vi "sub_main_vision.vi"(8 "error in":errorcluster) -> (0 "error out":errorcluster)   [LabVIEW 2019]
uses:
  <vilib>/vision/NI_Vision_Development_Module.lvlib
panel:
  out "강도 그래프":u8[][](graph)
  out "Image Pixels (U8)":u8[][](array[numeric])
  in  "Replace Value":sgl=1.0 format="%.2f"
  out "loop":i32
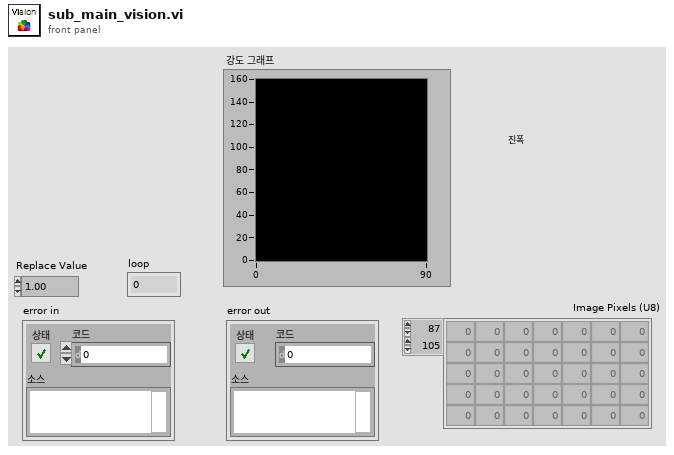
[diagram p1: front panel]
types:
  T1 = enum16{"none", "C920", "C922", "GT1290C", "MS LifeCam"}
  T2 = typedef "system_hw.ctl" = cluster{"AGV":enum16{"none", "ERP42", "ERP42mini", "Scout", "Ycar"}, "Lidar 1":enum16{"none", "VLP16", "TIM571", "RPLidar A2", "RPLidar A3"}, "Lidar 2":enum16{"none", "VLP16", "TIM571", "RPLidar A2", "RPLidar A3"}, "GPS":enum16{"none", "F9P", "M8P", "PwrPak7", "19X HVS"}, "Camera":enum16{"none", "C920", "C922", "GT1290C", "MS LifeCam"}, "Joystick":enum16{"none", "joystick"}}
  T3 = typedef "IMAQ Image.ctl" = refnum<image>
  T4 = cluster{"Clamp Settings":cluster{"Contrast":i32, "Filter width":i32, "Steepness":i32, "Subsampling Ratio":u32, "Show Search Area":bool, "Show Search Lines":bool, "Show Edges Found":bool, "Show Result":bool}, "Range":cluster{"Lower value":sgl, "Upper value":sgl}, "N of Erosion 1":i32, "N of Erosion 2":i32}
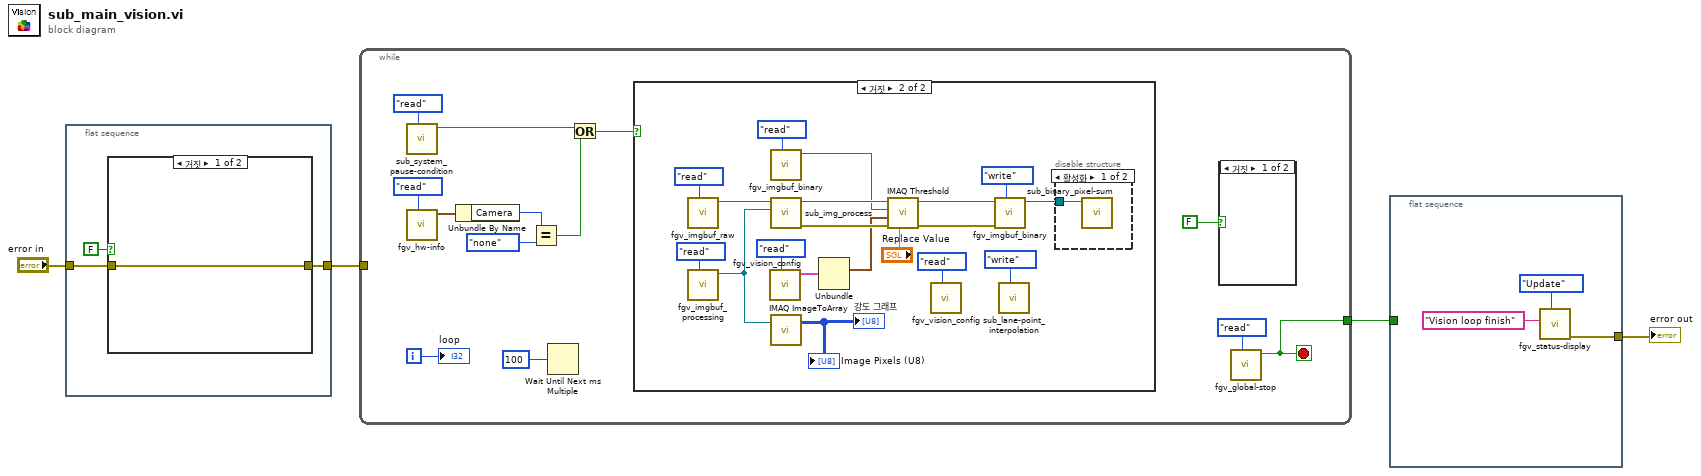
[diagram p0: block diagram]
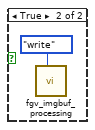
[diagram p2: hidden frame]
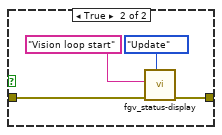
[diagram p5: hidden frame]
diagram:
  n1 = flat-sequence {
    tunnel: "error in" -> [w7]
    tunnel: [w6] -> w4
    frame #0 {
      n2 = case shown="거짓" FALSE {
        tunnel: w7 -> [w8 w10]
        tunnel: [w8 w9] -> w6
        frame False {
        }
        frame True {
          n3 = call "fgv_status-display.vi"("Mode"=enum16{"Initial", "Update", "Clear"}."Update", "error in"=w10, "title"="Vision loop start" ("String in 1")) -> ("error out"=w9:errorcluster)  [unwired: 8 in]
        }
      }
    }
  }
  n4 = while {
    tunnel: [w24] -> w1
    tunnel: w4 -> [_]
    i -> [w21]
    stop <- w24 stop-if-true
    n5 = call "sub_system_pause-condition.vi"("cmd"=enum16{"pause", "go", "read"}."read") -> ("pause"=w14:bool)  [unwired: 10 in]
    n6 = call "fgv_hw-info.vi"("cmd"=enum16{"write", "read"}."read") -> ("HW info out"=w18:T2)  [unwired: 10 in]
    n7 = Unbundle By Name(w18) -> ("Camera"=w17:T1)
    n8 = Equal?(x=w17, y=T1."none") -> (x = y?=w15:bool)
    n9 = Wait Until Next ms Multiple(millisecond multiple=u32 100 ("dt")) -> ()  [unwired: 1 out]
    n10 = Or(x=w14, y=w15) -> (x .or. y?=w13:bool)
    n11 = case shown="거짓" w13 {
      frame True {
      }
      frame False {
        n12 = call "fgv_imgbuf_raw.vi"("cmd"=enum16{"create", "close", "write", "read"}."read") -> ("Image"=w43:T3)  [unwired: 9 in, 1 out]
        n13 = call "fgv_imgbuf_processing.vi"("cmd"=enum16{"create", "close", "write", "read"}."read") -> ("Image"=w29:T3)  [unwired: 9 in, 1 out]
        n14 = call "fgv_vision_config.vi"("cmd"=enum16{"init", "read", "write"}."read") -> ("Vison cfg out"=w37:T4)  [unwired: 9 in, 1 out]
        n15 = call "fgv_imgbuf_binary.vi"("cmd"=enum16{"create", "close", "write", "read"}."read") -> ("raw image out"=w31:T3)  [unwired: 9 in, 1 out]
        n16 = call "sub_img_process.vi"("Green or Sat Plane"=w29, "Image Src"=w43) -> ("error out"=w39:errorcluster, "Image Dst Out"=w41:T3)  [unwired: 8 in]
        n17 = call "IMAQ ImageToArray"("Image"=w29) -> ("Image Pixels (U8)"=→"Image Pixels (U8)" →"강도 그래프":u8[][])  [unwired: 3 in, 4 out]
        n18 = Unbundle(w37) -> ("Range"=w35:cluster{"Lower value":sgl, "Upper value":sgl})  [unwired: 3 out]
        n19 = call "IMAQ Threshold"("Replace Value"="Replace Value", "error in (no error)"=w39, "Range"=w35, "Image Dst"=w31, "Image Src"=w41) -> ("error out"=w27:errorcluster, "Image Dst Out"=w28:T3)  [unwired: 5 in]
        n20 = call "fgv_vision_config.vi"("cmd"=enum16{"init", "read", "write"}."read") -> ()  [unwired: 9 in, 2 out]
        n21 = call "fgv_imgbuf_binary.vi"("cmd"=enum16{"create", "close", "write", "read"}."write", "error in"=w27, "raw Image in"=w28) -> ("raw image out"=w36:T3)  [unwired: 7 in, 1 out]
        n22 = call "sub_lane-point_interpolation.vi"("cmd"=enum16{"init", "read", "write"}."write") -> ()  [unwired: 7 in, 4 out]
        n23 = disable-structure shown="활성화" {
          disable-tunnel: w36 -> [w46 _]
          frame Enabled {
            n24 = call "sub_binary_pixel-sum.vi"("image buff"=w46) -> ()  [unwired: 9 in, 2 out]
          }
          frame Disabled {
          }
        }
      }
    }
    n25 = case shown="거짓" FALSE {
      frame False {
      }
      frame True {
        n26 = call "fgv_imgbuf_processing.vi"("cmd"=enum16{"create", "close", "write", "read"}."write") -> ()  [unwired: 9 in, 2 out]
      }
    }
    n27 = call "fgv_global-stop.vi"("cmd"=enum16{"init", "stop", "read"}."read") -> ("val_out"=w24:bool)  [unwired: 10 in]
    "loop" <- w21
  }
  n28 = flat-sequence {
    tunnel: w1 -> [_]
    tunnel: [w47] -> w3
    frame #0 {
      n29 = call "fgv_status-display.vi"("Mode"=enum16{"Initial", "Update", "Clear"}."Update", "title"="Vision loop finish" ("String in 1")) -> ("error out"=w47:errorcluster)  [unwired: 9 in]
    }
  }
  "error out" <- w3
